vi "Send VDH-RequestCalibration.vi"(7 "Message Priority (Normal)":T2=enum."Normal", 8 "error in (no error)":errorcluster, 10 "Calibration Type":T1=enum."Short", 11 "Message Enqueuer":refnum<class "Message Enqueuer.lvclass">) -> (0 "error out":errorcluster, 3 "Message Enqueuer out":refnum<class "Message Enqueuer.lvclass">)   [LabVIEW 2020, in "VDH-VNA_data_handler.lvlib" / "VDH-RequestCalibration Msg.lvclass"]
doc: "This VI sends the message to an actor."
uses:
  VDH-RequestCalibration Msg.lvclass
  <vilib>/ActorFramework/Message Enqueuer/Message Enqueuer.lvclass
  <vilib>/ActorFramework/Message Enqueuer/Message Priority.ctl
  VDH-VNA_data_handler/VDH-Calibration_enum.ctl
  C:/Program Files (x86)/National Instruments/LabVIEW 2020/vi.lib/ActorFramework/Message/Message.lvclass
  VDH-RequestCalibration Msg.lvclass/VDH-RequestCalibration Msg.ctl
  <vilib>/ActorFramework/Message Enqueuer/Message Enqueuer.lvclass/Message Enqueuer.ctl
  <vilib>/ActorFramework/Message Priority Queue/Priority Enqueue.vi
  VDH-VNA_data_handler/VDH-VNA_data_handler.lvclass
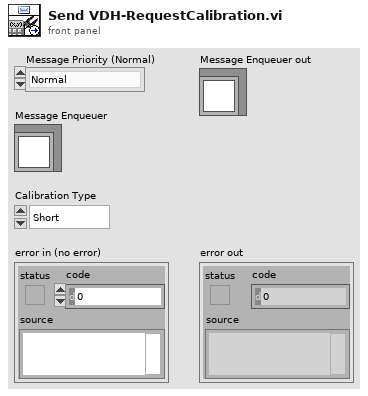
[diagram p1: front panel]
types:
  T1 = typedef "VDH-VNA_data_handler.lvlib/VDH-VNA_data_handler.lvclass/VDH-Calibration_enum.ctl" = enum16{"Non", "Short", "Open", "Load", "Through", "Permativity"}
  T2 = typedef "Actor Framework.lvlib/Message Enqueuer.lvclass/Message Priority.ctl" = enum16{"Low", "Normal", "High"}
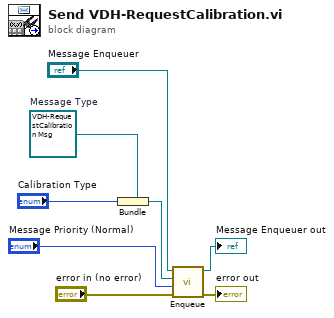
[diagram p0: block diagram]
diagram:
  w5 = refnum<class "VDH-RequestCalibration Msg.lvclass"> refnum  # Message Type
  n1 = Bundle(cluster=w5, "Calibration Type") -> (w4:refnum<class "VDH-RequestCalibration Msg.lvclass">)
  n2 = call <vilib>:"Enqueue.vi"("error in (no error)"="error in (no error)", "Message Priority (Normal)"="Message Priority (Normal)", "Message"=w4, "Message Enqueuer in"="Message Enqueuer") -> ("error out"=→"error out":errorcluster, "Message Enqueuer out"=→"Message Enqueuer out":refnum<class "Message Enqueuer.lvclass">)  [unwired: 6 in]
